vi "Teleop.vi"(10 "Match Info":T1={"Autonomous Elapsed Seconds"=0.0, "TeleOp Elapsed Seconds"=0.0, "Disabled Elapsed Seconds"=0.0, "Visited Autonomous"=FALSE, "Visited TeleOp"=FALSE, "Visited Disabled"=FALSE, "Autonomous Settings"={"Autonomous Style"=enum."Independent", "VI Refnum"=refnum}}, 11 "Call Context":T2) -> ()   [LabVIEW 2012]
doc: "This VI is called for each TeleOp packet received from the DS where the robot is not disabled. It is often used to read from the joysticks and update I/O or to update setpoints for timed control loops. It should complete and return within 20 milliseconds or it may miss DS packets."
uses:
  <vilib>/Rock Robotics/WPI/DriverStation/WPI_DriverStationDerivedRobotMode.ctl
  <vilib>/Rock Robotics/WPI/DriverStation/WPI_DriverStationMatch Info.ctl
  Robot Global Data.vi
  <vilib>/Rock Robotics/WPI/Joystick/WPI_JoystickGetSetRefNum.vi
  <vilib>/Rock Robotics/WPI/RobotDrive/WPI_RobotDriveGetSetRefNum.vi
panel:
  out "zAvit":dbl(graph)
  out "% OF RANGE":dbl(graph)
  out "Sensor Output":dbl(graph)
  out "angle zAvit":dbl
  out "Angle":u16
  in  "reset":bool
  out "in cannon":bool
  out "in flipper":bool
  out "middle":bool
  out "bottom":bool
  out "Conveyer belt joystick overwrite":dbl
  out "Shoot Motors":dbl
  out "Elevation":dbl
  out "Go Manual":bool
  out "auto shooting management":bool
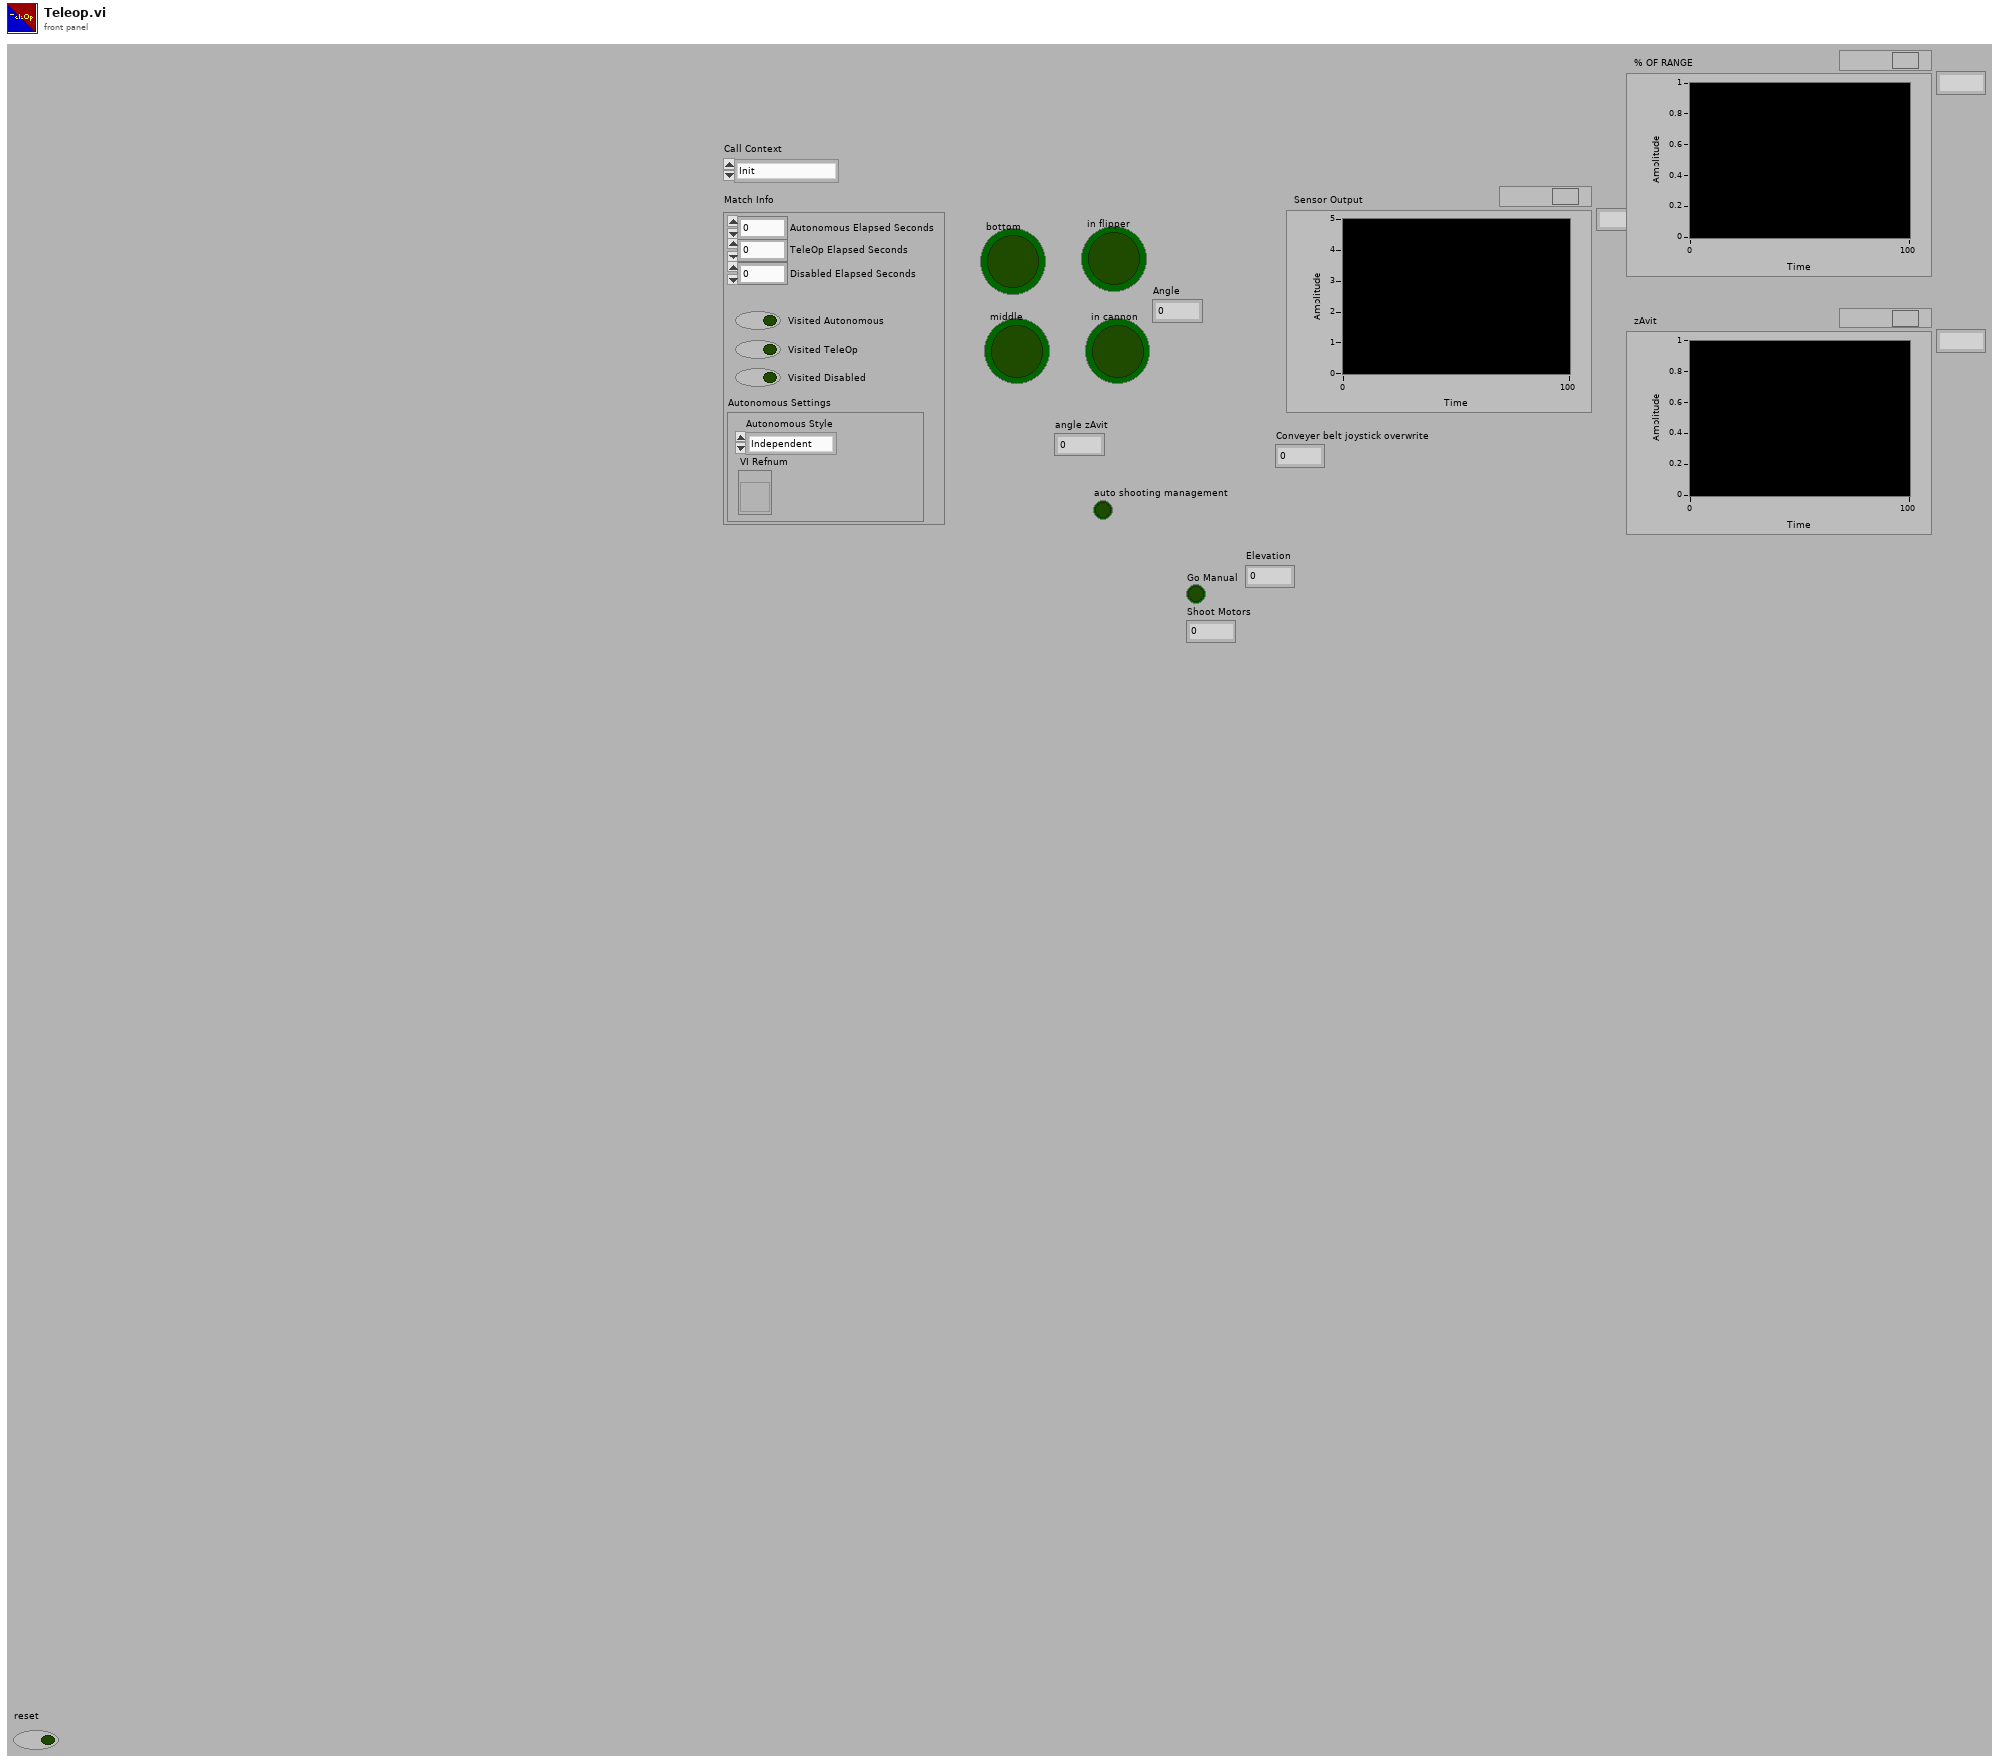
[diagram p1: front panel]
types:
  T1 = typedef "WPI_DriverStationMatch Info.ctl" = cluster{"Autonomous Elapsed Seconds":dbl, "TeleOp Elapsed Seconds":dbl, "Disabled Elapsed Seconds":dbl, "Visited Autonomous":bool, "Visited TeleOp":bool, "Visited Disabled":bool, "Autonomous Settings":cluster{"Autonomous Style":enum16{"Iterative", "Independent"}, "VI Refnum":refnum<vi>}}
  T2 = typedef "WPI_DriverStationDerivedRobotMode.ctl" = enum16{"Init", "Execute", "Stop"}
  T3 = typedef "WPI_ServoDeviceRef.ctl" = cluster{"DeviceStatus":errorcluster, "Digital Module":T4, "PWM Channel":T5, "DeadBand":T6}
  T4 = typedef "FPGA_TypedefDigitalModule.ctl" = enum16{"Digital Module 1", "Digital Module 2"}
  T5 = typedef "FPGA_DIOPWMChannel.ctl" = enum8{"PWM 1", "PWM 2", "PWM 3", "PWM 4", "PWM 5", "PWM 6", "PWM 7", "PWM 8", "PWM 9", "PWM 10", "Invalid"}
  T6 = typedef "WPI_PWMDeadband.ctl" = cluster{"Name":string, "maxPositivePwm":i32, "minPositivePwm":i32, "centerPwm":i32, "maxNegativePwm":i32, "minNegativePwm":i32, "angularRange":u16}
  T7 = typedef "WPI_AnalogChannelDevRef.ctl" = cluster{"DevStatus":errorcluster, "Analog Module":T8, "Analog Channel":T9}
  T8 = typedef "FPGA_TypedefAnalogModule.ctl" = enum16{"Analog Module 1", "Analog Module 2"}
  T9 = typedef "FPGA_AIChannel.ctl" = enum8{"AI 1", "AI 2", "AI 3", "AI 4", "AI 5", "AI 6", "AI 7", "AI 8", "Invalid"}
  T10 = typedef "WPI_JoystickDevRef.ctl" = cluster{"Device":T11}
  T11 = typedef "WPI_JoystickDeviceEnum.ctl" = enum16{"USB 1", "USB 2", "USB 3", "USB 4", "Kinect 1", "Kinect 2"}
  T12 = typedef "WPI_DigitalInputDevRef.ctl" = cluster{"DevStatus":errorcluster, "DIO Channel":T13, "Digital Module":T4}
  T13 = typedef "FPGA_DIOChannel.ctl" = enum8{"DIO 1", "DIO 2", "DIO 3", "DIO 4", "DIO 5", "DIO 6", "DIO 7", "DIO 8", "DIO 9", "DIO 10", "DIO 11", "DIO 12", "DIO 13", "DIO 14", "Invalid"}
  T14 = typedef "WPI_RobotDriveDevRef.ctl" = cluster{"DevStatus":errorcluster, "Motors[]":T15[], "Square Inputs":bool, "Max Output":dbl, "Isochronous":bool}
  T15 = typedef "WPI_MotorControlDeviceRef.ctl" = cluster{"DeviceStatus":errorcluster, "Type":enum16{"PWM", "CAN"}, "PWM":cluster{"Digital Module":T4, "PWM Channel":T5, "DeadBand":T6}, "CAN":cluster{"Device Number":u8, "Control Mode":T16, "Semaphore":T17, "Max Vout":dbl}, "Invert":bool, "TransformRef":T18, "InvTransformRef":T18}
  T16 = typedef "WPI_CANJaguar_ControlMode.ctl" = enum8{"Percent VBus", "Current", "Speed", "Position", "Voltage"}
  T17 = typedef "Semaphore RefNum" = refnum<k1>
  T18 = typedef "WPI_PWMTransform_ConPane.ctl" = refnum<vi>
  T19 = typedef "WPI_EncoderDevRef.ctl" = cluster{"DevStatus":errorcluster, "EncoderIndex":T20, "CounterIndex":T21, "DistancePerCount":dbl, "Decoding Type":T22}
  T20 = typedef "FPGA_EncoderIdx.ctl" = enum8{"Enc 0", "Enc 1", "Enc 2", "Enc 3", "Invalid"}
  T21 = typedef "FPGA_CounterCtrSystemIndex.ctl" = enum8{"Ctr 0", "Ctr 1", "Ctr 2", "Ctr 3", "Ctr 4", "Ctr 5", "Ctr 6", "Ctr 7", "Invalid"}
  T22 = typedef "WPI_EncoderType.ctl" = enum16{"1x", "2x", "4x"}
  T23 = typedef "WPI_RelayDevRef.ctl" = cluster{"DevStatus":errorcluster, "Relay Channel":T24, "Digital Module":T4, "Relay Direction":T25}
  T24 = typedef "FPGA_DIORelayChannel.ctl" = enum8{"Relay 1", "Relay 2", "Relay 3", "Relay 4", "Relay 5", "Relay 6", "Relay 7", "Relay 8", "Invalid"}
  T25 = typedef "WPI_RelayDirection.ctl" = enum16{"Both directions", "Forward only", "Reverse only"}
  T26 = typedef "WPI_RelayValue.ctl" = enum16{"Off", "On", "Forward", "Reverse"}
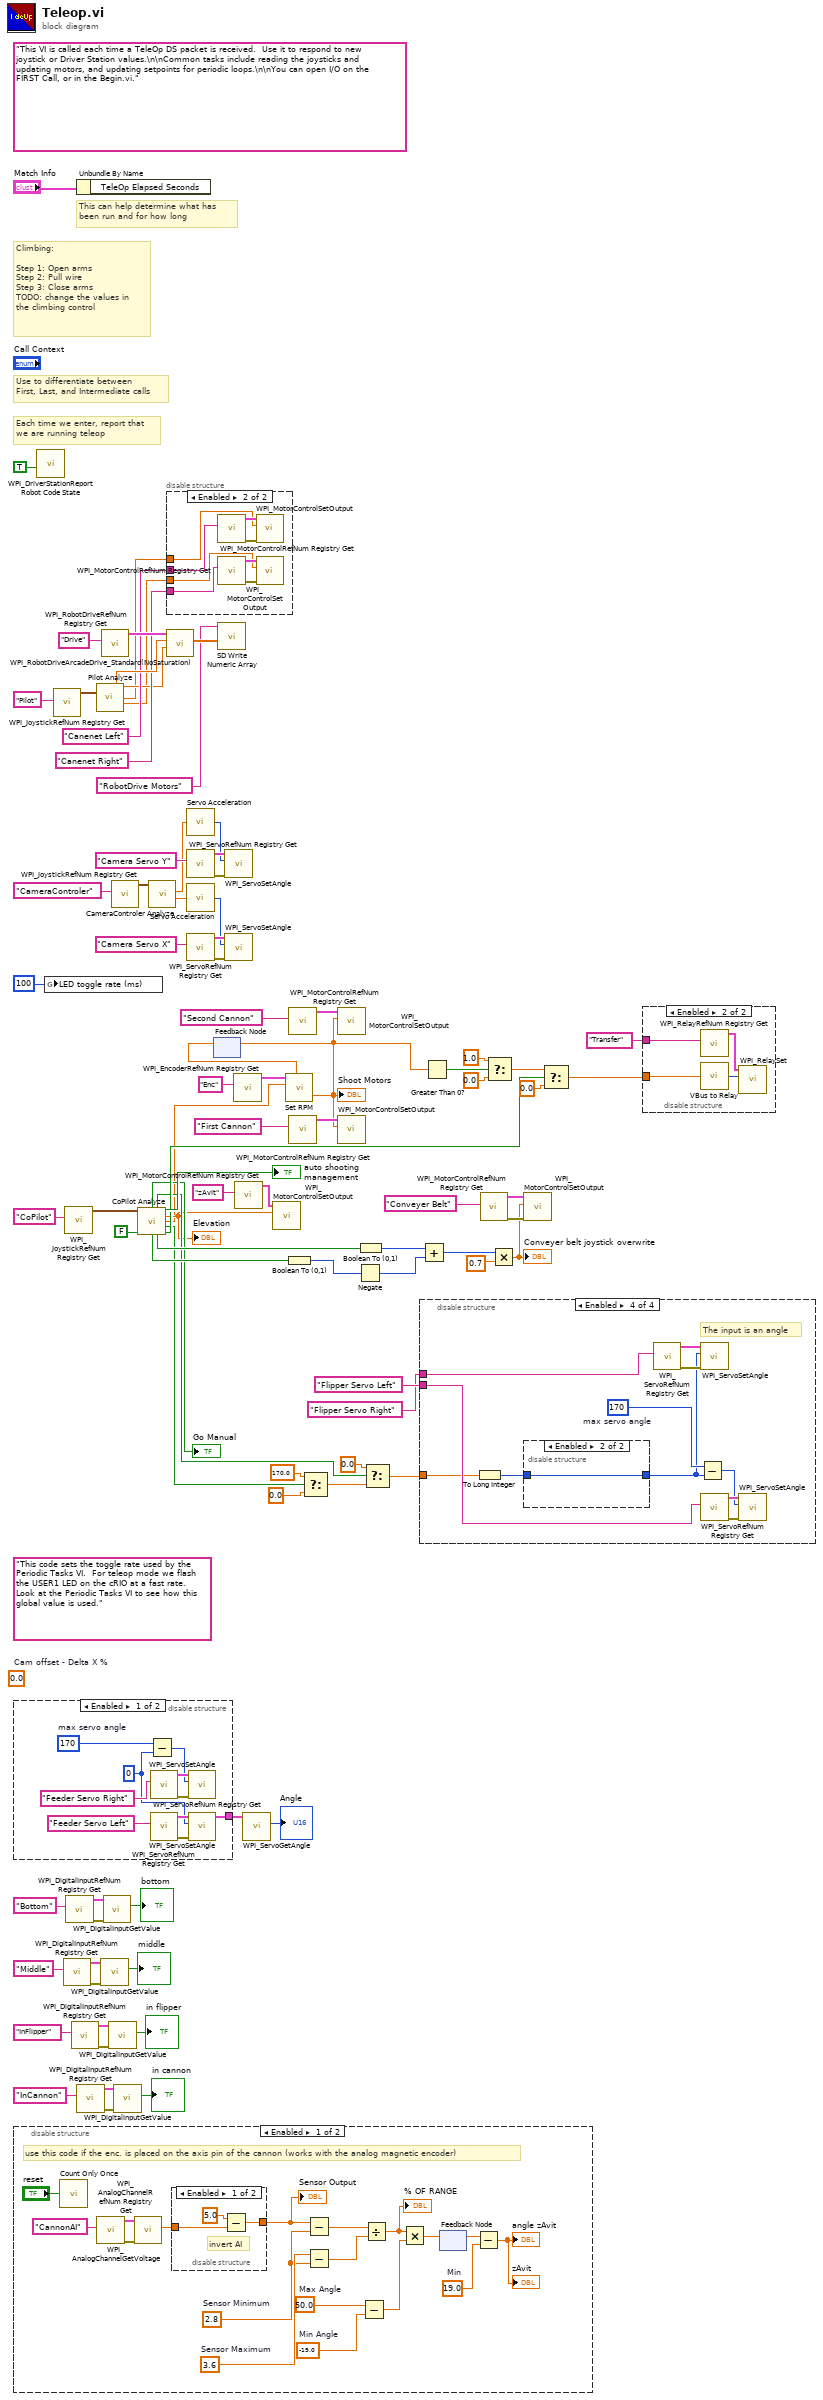
[diagram p0: block diagram]
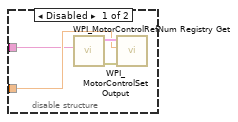
[diagram p5: hidden frame]
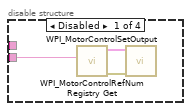
[diagram p6: hidden frame]
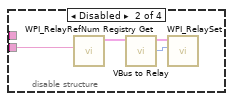
[diagram p7: hidden frame]
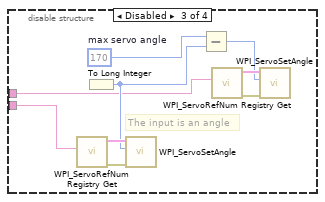
[diagram p8: hidden frame]
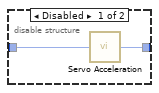
[diagram p9: hidden frame]
diagram:
  (unwired) 0.0  # Cam offset - Delta X %
  (unwired) "This code sets the toggle rate used by the Periodic Tasks VI.  For teleop mode we flash the USER1 LED on the cRIO at a fast rate.  Look at the Periodic Tasks VI to see how this global value is used."
  (unwired) "This VI is called each time a TeleOp DS packet is received.  Use it to respond to new joystick or Driver Station values.\n\nCommon tasks include reading the joysticks and updating motors, and updating setpoints for periodic loops.\n\nYou can open I/O on the FIRST Call, or in the Begin.vi."
  # "Climbing:\n\nStep 1: Open arms\nStep 2: Pull wire\nStep 3: Close arms\nTODO: change the values in \nthe climbing control"
  # "Each time we enter, report that\nwe are running teleop"
  # "Use to differentiate between\nFirst, Last, and Intermediate calls"
  # "This can help determine what has\nbeen run and for how long"
  n1 = disable-structure shown="Enabled" {
    disable-tunnel: [w91 _] -> w9
    frame Enabled {
      w92 = 0 ("number")
      w96 = 170  # max servo angle
      n2 = Subtract(x=w96, y=w92) -> (x-y=w93:i32)
      n3 = call <vilib>:"WPI_ServoRefNum Registry Get.vi"("refnum name"="Feeder Servo Right") -> ("error out"=w97:errorcluster, "ServoDeviceRef"=w98:T3)  [unwired: 9 in]
      n4 = call <vilib>:"WPI_ServoRefNum Registry Get.vi"("refnum name"="Feeder Servo Left") -> ("error out"=w99:errorcluster, "ServoDeviceRef"=w100:T3)  [unwired: 9 in]
      n5 = call <vilib>:"WPI_ServoSetAngle.vi"("error in (no error)"=w97, "Angle"=w93, "ServoDeviceRef"=w98) -> ()  [unwired: 7 in, 2 out]
      n6 = call <vilib>:"WPI_ServoSetAngle.vi"("error in (no error)"=w99, "Angle"=w92, "ServoDeviceRef"=w100) -> ("ServoDeviceRef"=w91:T3)  [unwired: 7 in, 1 out]
    }
    frame Disabled {
    }
  }
  n7 = disable-structure shown="Enabled" {
    frame Enabled {
      w104 = 2.8  # Sensor Minimum
      w105 = 3.6  # Sensor Maximum
      w108 = 19.0  # Min
      w112 = 50.0  # Max Angle
      w109 = -19.0  # Min Angle
      # "use this code if the enc. is placed on the axis pin of the cannon (works with the analog magnetic encoder)"
      n8 = call "Count Only Once.vi"("InValue"="reset") -> ()  [unwired: 1 out]
      n9 = call <vilib>:"WPI_AnalogChannelRefNum Registry Get.vi"("refnum name"="CannonAI") -> ("error out"=w115:errorcluster, "AIDeviceRef"=w117:T7)  [unwired: 9 in]
      n10 = call <vilib>:"WPI_AnalogChannelGetVoltage.vi"("error in (no error)"=w115, "AIDeviceRef"=w117) -> ("Voltage"=w116:dbl)  [unwired: 7 in, 2 out]
      n11 = disable-structure shown="Enabled" {
        disable-tunnel: w116 -> [w121 w122]
        disable-tunnel: [w120 w122] -> w113
        frame Enabled {
          # "invert AI"
          n12 = Subtract(x=5.0, y=w121) -> (x-y=w120:dbl)
        }
        frame Disabled {
        }
      }
      "Sensor Output" <- w113
      n13 = Subtract(x=w113, y=w104) -> (x-y=w102:dbl)
      n14 = Subtract(x=w105, y=w104) -> (x-y=w103:dbl)
      n15 = Subtract(x=w112, y=w109) -> (x-y=w111:dbl)
      n16 = Divide(x=w102, y=w103) -> (x/y=w110:dbl)
      "% OF RANGE" <- w110
      n17 = Multiply(x=w110, y=w111) -> (x*y=w107:dbl)
      n18 = feedback-in #1(w107) -> ()
      n19 = feedback #1() -> (w106:dbl)  [unwired: 1 in]
      n20 = Subtract(x=w106, y=w108) -> (x-y=→"angle zAvit" →"zAvit":dbl)
    }
    frame Disabled {
    }
  }
  n21 = call <vilib>:"WPI_DriverStationReport Robot Code State.vi"("TeleOp"=TRUE ("Autonomous")) -> ()  [unwired: 10 in, 1 out]
  n22 = global write "Robot Global Data.vi" "LED toggle rate (ms)"(u32 100 ("LED ms toggle rate")) -> ()
  n23 = call <vilib>:"WPI_JoystickRefNum Registry Get.vi"("refnum name"="Pilot") -> ("JoystickDevRef"=w86:T10)  [unwired: 1 in, 9 out]
  n24 = call <vilib>:"WPI_DigitalInputRefNum Registry Get.vi"("refnum name"="Middle") -> ("error out"=w23:errorcluster, "DigitalInputDevRef"=w24:T12)  [unwired: 9 in]
  n25 = call <vilib>:"WPI_JoystickRefNum Registry Get.vi"("refnum name"="CoPilot") -> ("JoystickDevRef"=w76:T10)  [unwired: 1 in, 9 out]
  n26 = call <vilib>:"WPI_DigitalInputRefNum Registry Get.vi"("refnum name"="Bottom") -> ("error out"=w27:errorcluster, "DigitalInputDevRef"=w26:T12)  [unwired: 9 in]
  n27 = call <vilib>:"WPI_DigitalInputRefNum Registry Get.vi"("refnum name"="InFlipper") -> ("error out"=w21:errorcluster, "DigitalInputDevRef"=w20:T12)  [unwired: 9 in]
  n28 = Unbundle By Name("Match Info") -> ()  [unwired: 1 out]
  n29 = call <vilib>:"WPI_DigitalInputRefNum Registry Get.vi"("refnum name"="InCannon") -> ("error out"=w17:errorcluster, "DigitalInputDevRef"=w18:T12)  [unwired: 9 in]
  n30 = call "Pilot Analyze.vi"("JoystickDevRef"=w86) -> ("x"=w80:dbl, "y"=w7:dbl, "Canenet L"=w6:dbl, "Canenet R"=w5:dbl)  [unwired: 8 in, 3 out]
  n31 = call <vilib>:"WPI_DigitalInputGetValue.vi"("error in (no error)"=w23, "DigitalInputDevRef"=w24) -> ("Value"=→"middle":bool)  [unwired: 7 in, 2 out]
  n32 = call <vilib>:"WPI_RobotDriveRefNum Registry Get.vi"("refnum name"="Drive") -> ("RobotDriveDevRef"=w82:T14)  [unwired: 1 in, 9 out]
  n33 = call <vilib>:"WPI_DigitalInputGetValue.vi"("error in (no error)"=w27, "DigitalInputDevRef"=w26) -> ("Value"=→"bottom":bool)  [unwired: 7 in, 2 out]
  n34 = call <vilib>:"WPI_DigitalInputGetValue.vi"("error in (no error)"=w21, "DigitalInputDevRef"=w20) -> ("Value"=→"in flipper":bool)  [unwired: 7 in, 2 out]
  n35 = call <vilib>:"WPI_JoystickRefNum Registry Get.vi"("refnum name"="CameraControler") -> ("JoystickDevRef"=w78:T10)  [unwired: 1 in, 9 out]
  n36 = call <vilib>:"WPI_DigitalInputGetValue.vi"("error in (no error)"=w17, "DigitalInputDevRef"=w18) -> ("Value"=→"in cannon":bool)  [unwired: 7 in, 2 out]
  n37 = call "CoPilot Analyze.vi"("JoystickDevRef"=w76, "Climbing Manual Enabled"=FALSE) -> ("Go Manual"=→"Go Manual":bool, "Flipper Min"=w34:bool, "auto shooting management"=→"auto shooting management":bool, "Elevation"=w10:dbl, "Shoot Motors"=w1:dbl, "Flipper Max"=w37:bool, "conveyer belt down"=w73:bool, "conveyer belt up"=w74:bool, "La Fire at will?"=w42:bool)  [unwired: 5 in]
  "Elevation" <- w10
  n38 = call "CameraControler Analyze.vi"("JoystickDevRef"=w78) -> ("axis 3 (rotation)"=w50:dbl, "Y"=w30:dbl)  [unwired: 5 in, 4 out]
  n39 = disable-structure shown="Enabled" {
    disable-tunnel: "Canenet Right" ("refnum name") -> [_ w126]
    disable-tunnel: "Canenet Left" ("refnum name") -> [_ w125]
    disable-tunnel: w6 -> [_ w124]
    disable-tunnel: w5 -> [_ w123]
    frame Disabled {
    }
    frame Enabled {
      n40 = call <vilib>:"WPI_MotorControlRefNum Registry Get.vi"("refnum name"=w125) -> ("error out"=w127:errorcluster, "MotorControlDevRef"=w128:T15)  [unwired: 9 in]
      n41 = call <vilib>:"WPI_MotorControlRefNum Registry Get.vi"("refnum name"=w126) -> ("error out"=w130:errorcluster, "MotorControlDevRef"=w129:T15)  [unwired: 9 in]
      n42 = call <vilib>:"WPI_MotorControlSetOutput.vi"("error in (no error)"=w127, "Output"=w124, "MotorControlDevRef"=w128) -> ()  [unwired: 6 in, 3 out]
      n43 = call <vilib>:"WPI_MotorControlSetOutput.vi"("error in (no error)"=w130, "Output"=w123, "MotorControlDevRef"=w129) -> ()  [unwired: 6 in, 3 out]
    }
  }
  n44 = call <vilib>:"WPI_RobotDriveArcadeDrive_Standard(NoSaturation).vi"("Y axis value"=w7, "X axis value"=w80, "RobotDriveDevRef"=w82) -> ("Motor Values"=w84:dbl[])  [unwired: 1 in, 7 out]
  n45 = call "Servo Acceleration.vi"("Angle get"=w30) -> ("Angle Set"=w48:i32)  [unwired: 4 in]
  n46 = call <vilib>:"WPI_ServoRefNum Registry Get.vi"("refnum name"="Camera Servo Y") -> ("error out"=w64:errorcluster, "ServoDeviceRef"=w63:T3)  [unwired: 9 in]
  n47 = call "Servo Acceleration.vi"("Angle get"=w50) -> ("Angle Set"=w49:i32)  [unwired: 4 in]
  n48 = call <vilib>:"WPI_ServoRefNum Registry Get.vi"("refnum name"="Camera Servo X") -> ("error out"=w61:errorcluster, "ServoDeviceRef"=w62:T3)  [unwired: 9 in]
  n49 = feedback #2() -> (w4:dbl)  [unwired: 1 in]
  n50 = call <vilib>:"SD Write Numeric Array.vi"("Numeric Array"=w84, "Name"="RobotDrive Motors") -> ()  [unwired: 8 in, 2 out]
  n51 = call <vilib>:"WPI_ServoSetAngle.vi"("error in (no error)"=w64, "Angle"=w48, "ServoDeviceRef"=w63) -> ()  [unwired: 7 in, 2 out]
  n52 = call <vilib>:"WPI_ServoSetAngle.vi"("error in (no error)"=w61, "Angle"=w49, "ServoDeviceRef"=w62) -> ()  [unwired: 7 in, 2 out]
  n53 = call <vilib>:"WPI_EncoderRefNum Registry Get.vi"("refnum name"="Enc") -> ("EncoderDevRef"=w3:T19)  [unwired: 9 in, 1 out]
  n54 = call <vilib>:"WPI_MotorControlRefNum Registry Get.vi"("refnum name"="zAvit") -> ("MotorControlDevRef"=w59:T15)  [unwired: 9 in, 1 out]
  n55 = call <vilib>:"WPI_ServoGetAngle.vi"("ServoDeviceRef"=w9) -> ("Angle"=→"Angle":u16)  [unwired: 7 in, 2 out]
  n56 = call <vilib>:"WPI_MotorControlSetOutput.vi"("Output"=w10, "MotorControlDevRef"=w59) -> ()  [unwired: 7 in, 3 out]
  n57 = call "Set RPM.vi"("EncoderDevRef"=w3, "Set Point RPM"=w1, "Previous Vbus"=w4) -> ("Vbus Out"=w2:dbl)  [unwired: 2 in, 1 out]
  "Shoot Motors" <- w2
  n58 = feedback-in #2(w2) -> ()
  n59 = Boolean To (0,1)(Boolean=w73) -> (0, 1=w72:i16)
  n60 = call <vilib>:"WPI_MotorControlRefNum Registry Get.vi"("refnum name"="Second Cannon") -> ("MotorControlDevRef"=w55:T15)  [unwired: 9 in, 1 out]
  n61 = call <vilib>:"WPI_MotorControlRefNum Registry Get.vi"("refnum name"="First Cannon") -> ("MotorControlDevRef"=w56:T15)  [unwired: 9 in, 1 out]
  n62 = Select(t=170.0, s=w37, f=0.0) -> (s? t:f=w33:dbl)
  n63 = call <vilib>:"WPI_MotorControlSetOutput.vi"("Output"=w2, "MotorControlDevRef"=w55) -> ()  [unwired: 7 in, 3 out]
  n64 = call <vilib>:"WPI_MotorControlSetOutput.vi"("Output"=w2, "MotorControlDevRef"=w56) -> ()  [unwired: 7 in, 3 out]
  n65 = Boolean To (0,1)(Boolean=w74) -> (0, 1=w70:i16)
  n66 = Negate(x=w72) -> (-x=w71:i16)
  n67 = Select(t=0.0, s=w34, f=w33) -> (s? t:f=w31:dbl)
  n68 = disable-structure shown="Enabled" {
    disable-tunnel: "Flipper Servo Left" ("refnum name") -> [w131 w135 w145 w151]
    disable-tunnel: "Flipper Servo Right" ("refnum name") -> [_ _ w137 w150]
    disable-tunnel: w31 -> [_ _ _ w149]
    frame Disabled {
      n69 = call <vilib>:"WPI_MotorControlRefNum Registry Get.vi"("refnum name"=w131) -> ("error out"=w133:errorcluster, "MotorControlDevRef"=w132:T15)  [unwired: 9 in]
      n70 = call <vilib>:"WPI_MotorControlSetOutput.vi"("error in (no error)"=w133, "MotorControlDevRef"=w132) -> ()  [unwired: 7 in, 3 out]
    }
    frame Disabled {
      n71 = call <vilib>:"WPI_RelayRefNum Registry Get.vi"("refnum name"=w135) -> ("RelayDevRef"=w134:T23)  [unwired: 9 in, 1 out]
      n72 = call "VBus to Relay.vi"() -> ("RelayValue"=w136:T26)  [unwired: 4 in]
      n73 = call <vilib>:"WPI_RelaySet.vi"("RelayValue"=w136, "RelayDevRef"=w134) -> ()  [unwired: 8 in, 2 out]
    }
    frame Disabled {
      w140 = 170  # max servo angle
      # "The input is an angle"
      n74 = call <vilib>:"WPI_ServoRefNum Registry Get.vi"("refnum name"=w145) -> ("error out"=w143:errorcluster, "ServoDeviceRef"=w144:T3)  [unwired: 9 in]
      n75 = To Long Integer() -> (32bit integer=w139:i32)  [unwired: 1 in]
      n76 = call <vilib>:"WPI_ServoSetAngle.vi"("error in (no error)"=w143, "Angle"=w139, "ServoDeviceRef"=w144) -> ()  [unwired: 7 in, 2 out]
      n77 = Subtract(x=w140, y=w139) -> (x-y=w138:i32)
      n78 = call <vilib>:"WPI_ServoRefNum Registry Get.vi"("refnum name"=w137) -> ("error out"=w142:errorcluster, "ServoDeviceRef"=w141:T3)  [unwired: 9 in]
      n79 = call <vilib>:"WPI_ServoSetAngle.vi"("error in (no error)"=w142, "Angle"=w138, "ServoDeviceRef"=w141) -> ()  [unwired: 7 in, 2 out]
    }
    frame Enabled {
      w152 = 170  # max servo angle
      # "The input is an angle"
      n80 = To Long Integer(number=w149) -> (32bit integer=w148:i32)
      n81 = disable-structure shown="Enabled" {
        disable-tunnel: w148 -> [w158 w159]
        disable-tunnel: [w157 w159] -> w147
        frame Disabled {
          n82 = call "Servo Acceleration.vi"("Angle get"=w158) -> ("Angle Set"=w157:i32)  [unwired: 4 in]
        }
        frame Enabled {
        }
      }
      n83 = call <vilib>:"WPI_ServoRefNum Registry Get.vi"("refnum name"=w150) -> ("error out"=w155:errorcluster, "ServoDeviceRef"=w156:T3)  [unwired: 9 in]
      n84 = Subtract(x=w152, y=w147) -> (x-y=w146:i32)
      n85 = call <vilib>:"WPI_ServoSetAngle.vi"("error in (no error)"=w155, "Angle"=w147, "ServoDeviceRef"=w156) -> ()  [unwired: 7 in, 2 out]
      n86 = call <vilib>:"WPI_ServoRefNum Registry Get.vi"("refnum name"=w151) -> ("error out"=w154:errorcluster, "ServoDeviceRef"=w153:T3)  [unwired: 9 in]
      n87 = call <vilib>:"WPI_ServoSetAngle.vi"("error in (no error)"=w154, "Angle"=w146, "ServoDeviceRef"=w153) -> ()  [unwired: 7 in, 2 out]
    }
  }
  n88 = Add(x=w70, y=w71) -> (x+y=w68:i16)
  n89 = Greater Than 0?(x=w2) -> (x > 0?=w44:bool)
  n90 = call <vilib>:"WPI_MotorControlRefNum Registry Get.vi"("refnum name"="Conveyer Belt") -> ("error out"=w54:errorcluster, "MotorControlDevRef"=w53:T15)  [unwired: 9 in]
  n91 = Select(t=1.0, s=w44, f=0.0) -> (s? t:f=w43:dbl)
  n92 = Multiply(x=w68, y=0.7) -> (x*y=w51:dbl)
  "Conveyer belt joystick overwrite" <- w51
  n93 = call <vilib>:"WPI_MotorControlSetOutput.vi"("error in (no error)"=w54, "Output"=w51, "MotorControlDevRef"=w53) -> ()  [unwired: 6 in, 3 out]
  n94 = Select(t=w43, s=w42, f=0.0) -> (s? t:f=w41:dbl)
  n95 = disable-structure shown="Enabled" {
    disable-tunnel: w41 -> [w161 w164]
    disable-tunnel: "Transfer" ("refnum name") -> [w160 w166]
    frame Disabled {
      n96 = call <vilib>:"WPI_MotorControlRefNum Registry Get.vi"("refnum name"=w160) -> ("error out"=w163:errorcluster, "MotorControlDevRef"=w162:T15)  [unwired: 9 in]
      n97 = call <vilib>:"WPI_MotorControlSetOutput.vi"("error in (no error)"=w163, "Output"=w161, "MotorControlDevRef"=w162) -> ()  [unwired: 6 in, 3 out]
    }
    frame Enabled {
      n98 = call <vilib>:"WPI_RelayRefNum Registry Get.vi"("refnum name"=w166) -> ("RelayDevRef"=w165:T23)  [unwired: 9 in, 1 out]
      n99 = call "VBus to Relay.vi"("Motor VBus"=w164) -> ("RelayValue"=w167:T26)  [unwired: 3 in]
      n100 = call <vilib>:"WPI_RelaySet.vi"("RelayValue"=w167, "RelayDevRef"=w165) -> ()  [unwired: 8 in, 2 out]
    }
  }
